vi "project test.vi"() -> ()   [LabVIEW 2018]
uses:
  Projects/1259_usbComm/#include/Global_usbComm.vi
panel:
  out "standard labviewdbupload":string
  out "standard notepad":string
  out "Test Log":string
  out "Goodbye!":picture
  out "refnum out":refnum<file>
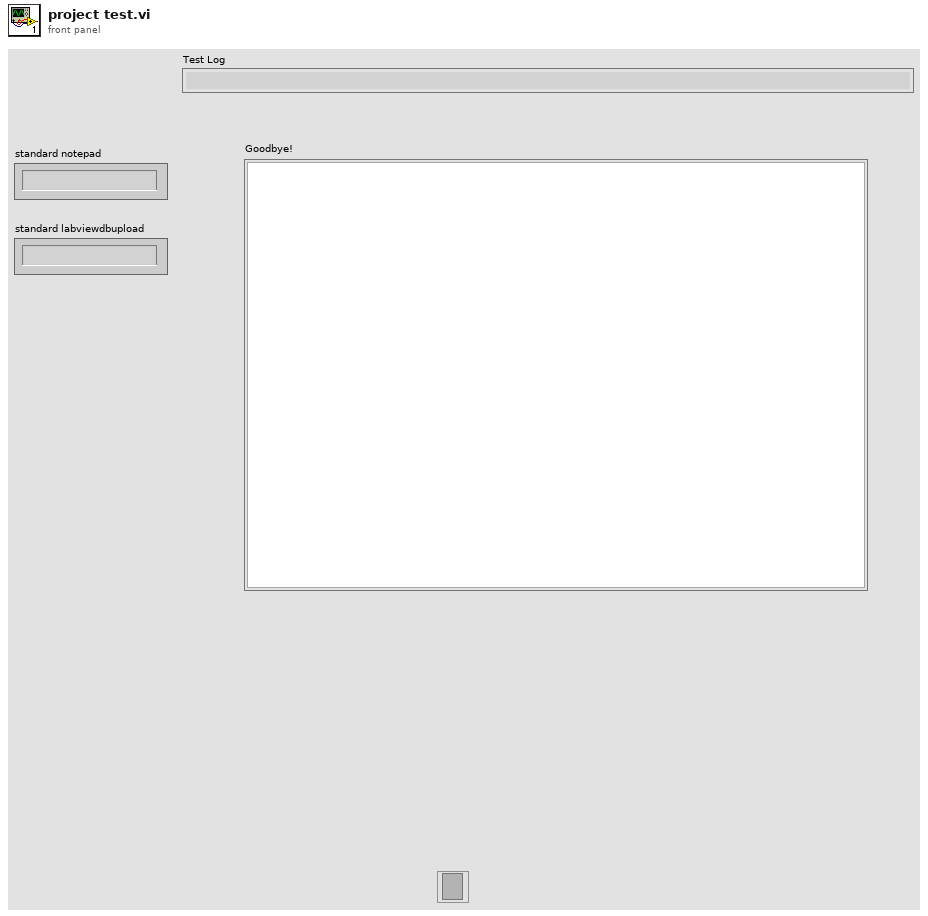
[diagram p1: front panel]
types:
  T1 = enum32{"Interactive applications", "Built-in command line utilities", "Executable command line utilities"}
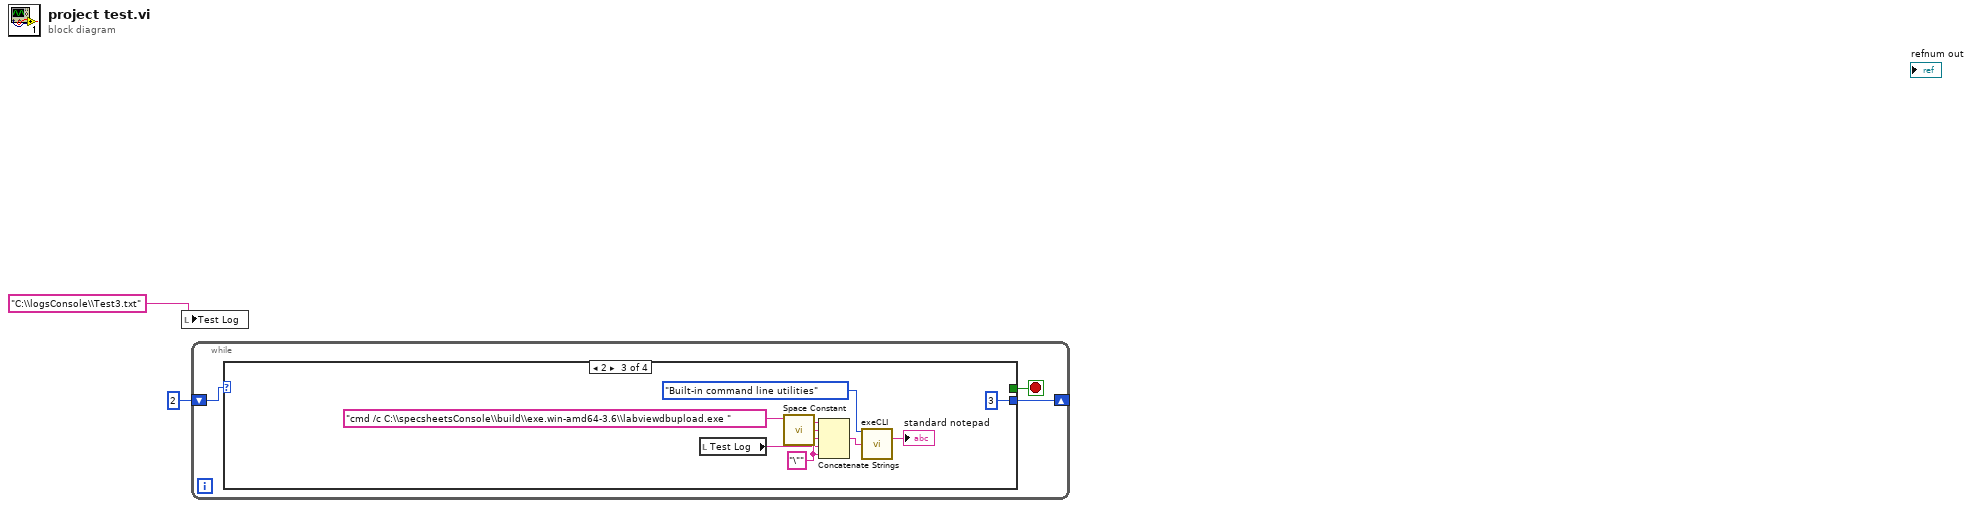
[diagram p0: block diagram]
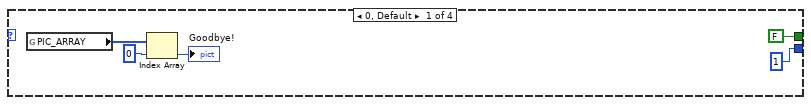
[diagram p2: hidden frame]
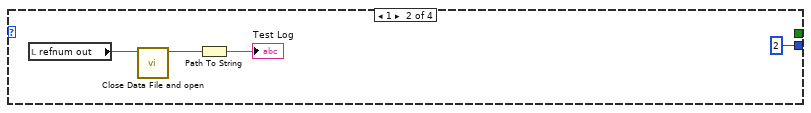
[diagram p3: hidden frame]
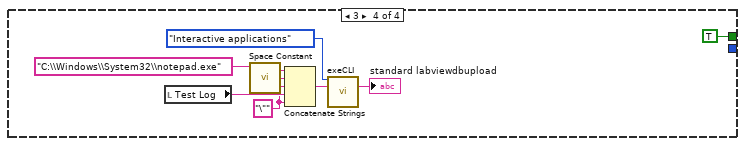
[diagram p4: hidden frame]
diagram:
  n1 = local write "Test Log"("C:\\logsConsole\\Test3.txt" ("String")) -> ()
  n2 = while {
    shift-right: [w3] -> _
    shift-left: 2 -> [w5]
    stop <- w4 stop-if-true
    n3 = case shown="2" w5 {
      tunnel: [FALSE _ _ TRUE] -> w4
      tunnel: [1 2 3 _] -> w3
      frame 0, Default {
        n4 = global read "Global_usbComm.vi" "PIC_ARRAY"() -> (w10:picture[])
        n5 = Index Array(array=w10, index=0) -> (element=→"Goodbye!":picture)
      }
      frame 1 {
        n6 = local read "refnum out"() -> (w14:refnum<file>)
        n7 = call "Close Data File and open.vi"("File Refnum In"=w14) -> ("path"=w13:path)  [unwired: 9 in, 1 out]
        n8 = Path To String(path=w13) -> (string=→"Test Log":string)
      }
      frame 2 {
        w17 = "\""
        n9 = local read "Test Log"() -> (w16:string)
        n10 = call <vilib>:"Space Constant.vi"() -> ("String"=w22:string)
        n11 = Concatenate Strings("cmd /c C:\\specsheetsConsole\\build\\exe.win-amd64-3.6\\labviewdbupload.exe ", w22, w17, w16, w17) -> (w15:string)
        n12 = call "exeCLI.vi"("Tab Control"=T1."Built-in command line utilities", "command line (built-in)"=w15) -> ("standard error"=→"standard notepad":string)  [unwired: 11 in, 2 out]
      }
      frame 3 {
        w24 = "\""
        n13 = local read "Test Log"() -> (w25:string)
        n14 = call <vilib>:"Space Constant.vi"() -> ("String"=w29:string)
        n15 = Concatenate Strings("C:\\Windows\\System32\\notepad.exe" ("Command"), w29, w24, w25, w24) -> (w30:string)
        n16 = call "exeCLI.vi"("Tab Control"=T1."Interactive applications", "command line (interactive)"=w30) -> ("standard error"=→"standard labviewdbupload":string)  [unwired: 11 in, 2 out]
      }
    }
  }
